vi "Double to Data Type.vi"(8 "error in (no error)":errorcluster, 11 "Double":dbl) -> (0 "error out":errorcluster, 3 "Boolean out":refnum<class "Double.lvclass">)   [LabVIEW 2019, in "Double.lvclass"]
uses:
  <vilib>/gpm_packages/@cs/data-type-serializer/source/Double/Double.lvclass
  <vilib>/gpm_packages/@cs/data-type-serializer/source/Double/Double.lvclass/Double.ctl
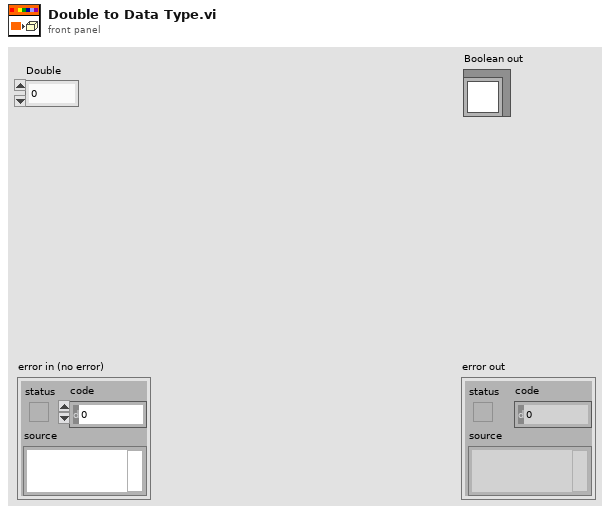
[diagram p1: front panel]
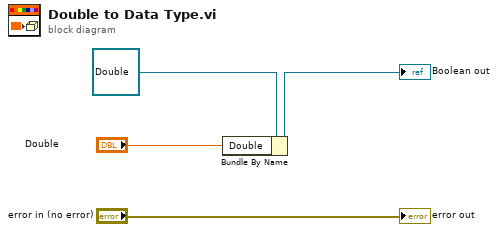
[diagram p0: block diagram]
diagram:
  n1 = Bundle By Name(cluster=refnum<class "Double.lvclass"> refnum ("Boolean in"), "Double"="Double") -> (→"Boolean out":refnum<class "Double.lvclass">)
  "error out" <- "error in (no error)"
